vi "Pitstop.vi"(8 "Robot in":T1, 9 "robos":u32[](array[numeric]), 10 "IA State Input":T3={"our_robots"=[], "enemy_robots"=[], "balls"=[], "geometry"={"line_width"=0, "field_length"=0, "field_width"=0, "boundary_width"=0, "referee_width"=0, "goal_width"=0, "goal_depth"=0, "goal_wall_width"=0, "center_circle_radius"=0, "defense_radius"=0, "defense_stretch"=0, "free_kick_from_defense_dist"=0, "penalty_spot_from_field_line_dist"=0, "penalty_line_from_spot_dist"=0}, "IA Judge"={"stage"="", "command"="", "our_goalie_id"=0.0, "enemy_goalie_id"=0.0, "command\nenum"=enum."Halt", "Time"=enum."Azul"}, "Received Timestamp"=timestamp(0 s since 1904-01-01), "Events"={"Touch"=FALSE, "Ball out"=FALSE, "id touch"=0.0, "Ball out of \nVision"=FALSE, "Ball inside \nGoalie area"=FALSE, "Robot not responding"=FALSE, "Robots responding status"=[1.0, 1.0, 1.0, 1.0, 1.0, 1.0]}}) -> (1 "Robot out":T1)   [LabVIEW 2016]
uses:
  Core/AI Input.ctl
  Core/AI Robot.ctl
  Functions Enum.ctl
  Core/AI Ball.ctl
  Core/Field Size.ctl
  Core/AI Judge.ctl
  Command Enum.ctl
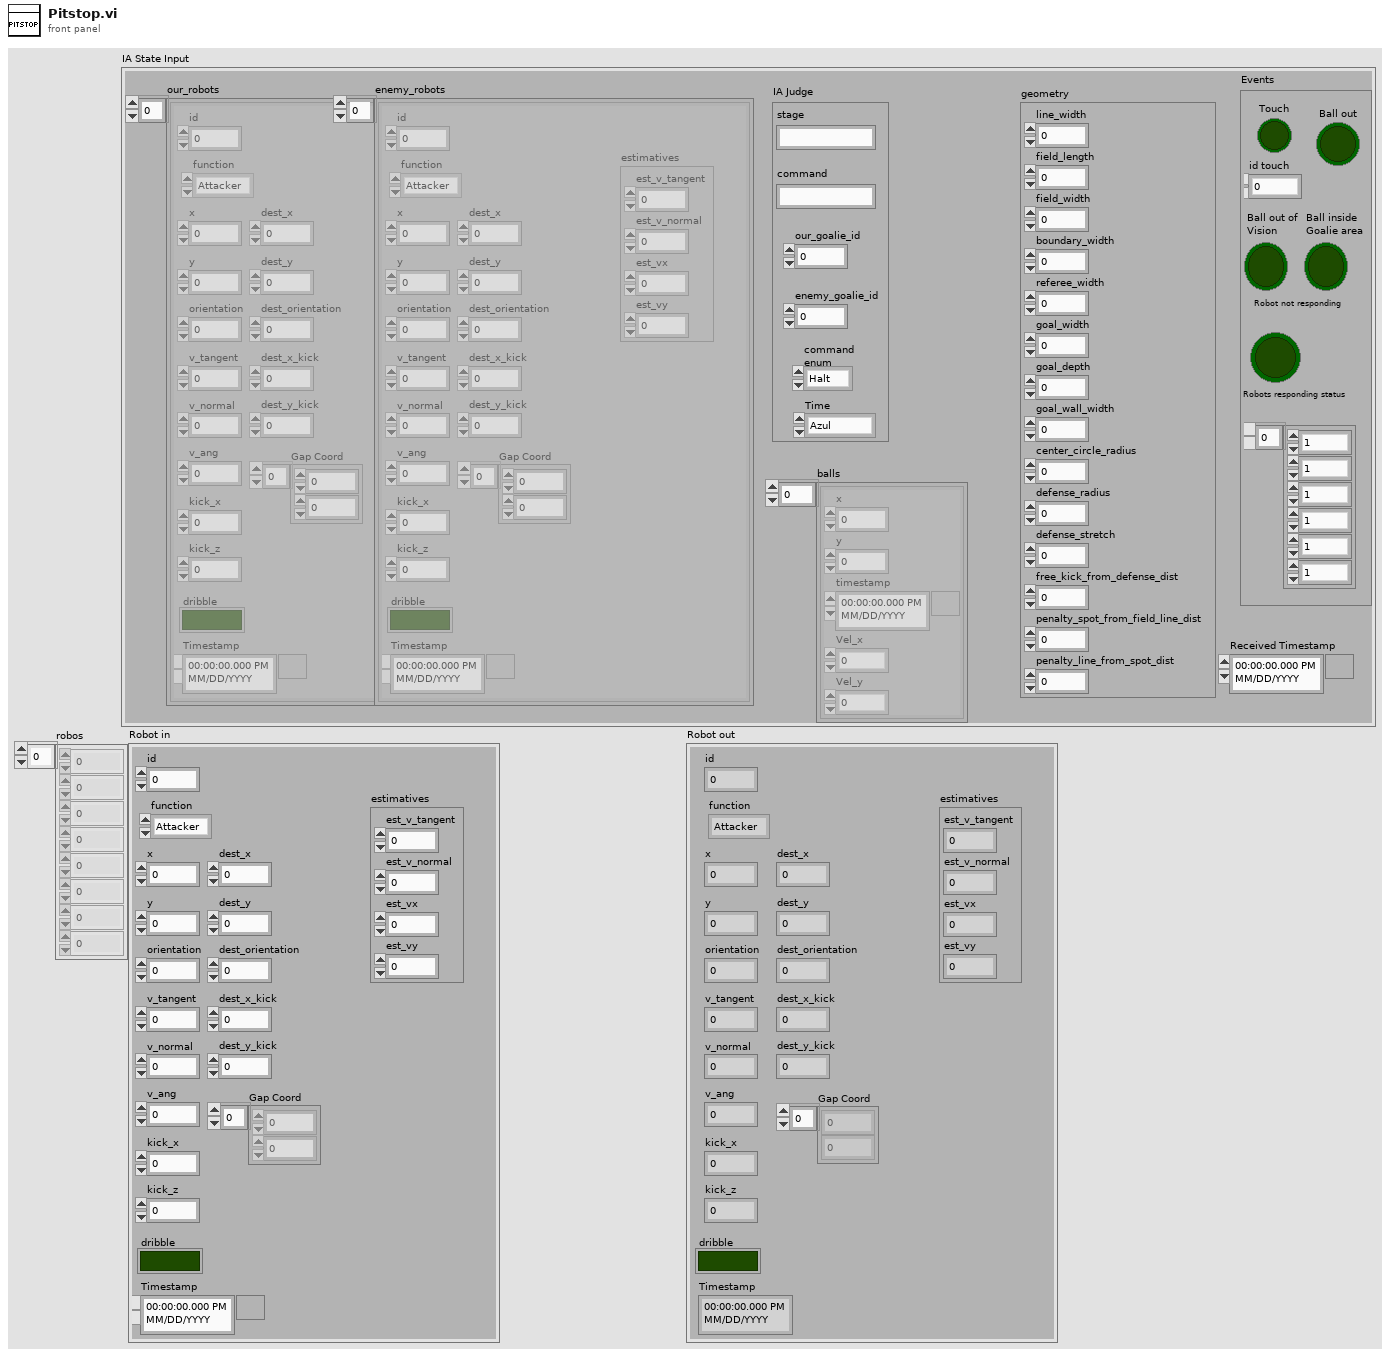
[diagram p1: front panel]
types:
  T1 = typedef "AI Robot.ctl" = cluster{"id":u32, "function":T2, "x":dbl, "y":dbl, "orientation":dbl, "v_tangent":dbl, "v_normal":dbl, "v_ang":dbl, "kick_x":dbl, "kick_z":dbl, "dribble":bool, "Timestamp":timestamp, "dest_x":dbl, "dest_y":dbl, "dest_orientation":dbl, "estimatives":cluster{"est_v_tangent":dbl, "est_v_normal":dbl, "est_vx":dbl, "est_vy":dbl}, "dest_x_kick":dbl, "dest_y_kick":dbl, "Gap Coord":dbl[]}
  T2 = typedef "Functions Enum.ctl" = enum16{"Attacker", "Goalie", "Defender", "Striker", "Goto 0", "Dummy", "Kicker", "ZigZag"}
  T3 = typedef "AI Input.ctl" = cluster{"our_robots":T1[], "enemy_robots":T1[], "balls":T4[], "geometry":T5, "IA Judge":T6, "Received Timestamp":timestamp, "Events":cluster{"Touch":bool, "Ball out":bool, "id touch":dbl, "Ball out of \nVision":bool, "Ball inside \nGoalie area":bool, "Robot not responding":bool, "Robots responding status":dbl[]}}
  T4 = typedef "AI Ball.ctl" = cluster{"x":dbl, "y":dbl, "timestamp":timestamp, "Vel_x":dbl, "Vel_y":dbl}
  T5 = typedef "Field Size.ctl" = cluster{"line_width":u32, "field_length":u32, "field_width":u32, "boundary_width":u32, "referee_width":u32, "goal_width":u32, "goal_depth":u32, "goal_wall_width":u32, "center_circle_radius":u32, "defense_radius":u32, "defense_stretch":u32, "free_kick_from_defense_dist":u32, "penalty_spot_from_field_line_dist":u32, "penalty_line_from_spot_dist":u32}
  T6 = typedef "AI Judge.ctl" = cluster{"stage":string, "command":string, "our_goalie_id":dbl, "enemy_goalie_id":dbl, "command\nenum":T7, "Time":enum16{"Azul", "Amarelo"}}
  T7 = typedef "Command Enum.ctl" = enum16{"Halt", "Stop", "Force Start", "PKA Normal Start", "Prepare Kickoff Ally", "PKE Normal Start", "Prepare Kickoff Enemy", "Prepare Penalty Ally", "PPA Normal Start", "Prepare Penalty Enemy", "PPE Normal Start", "Direct Free Enemy", "Direct Free Ally", "Indirect Free Enemy", "Indirect Free Ally", "Timeout Enemy", "Timeout Ally", "Goal Enemy", "Goal Ally", "Ball Placement Enemy", "Ball Placement Ally", "None"}
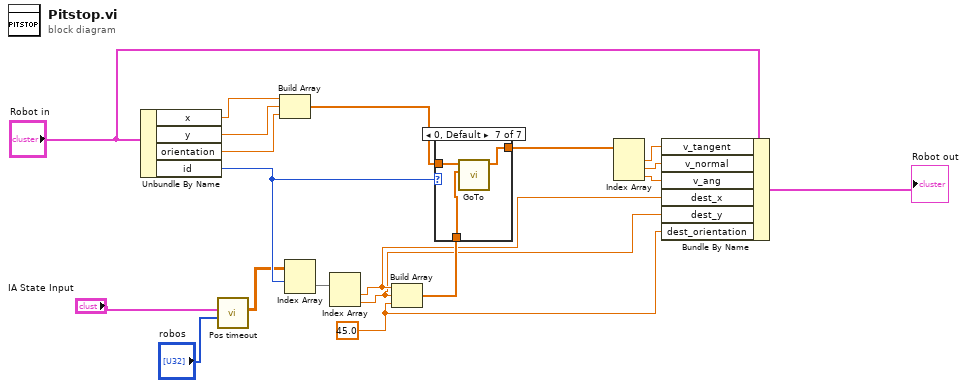
[diagram p0: block diagram]
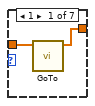
[diagram p2: hidden frame]
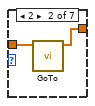
[diagram p3: hidden frame]
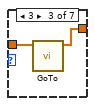
[diagram p4: hidden frame]
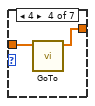
[diagram p5: hidden frame]
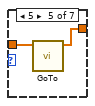
[diagram p6: hidden frame]
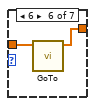
[diagram p7: hidden frame]
diagram:
  w4 = 45.0 ("element")
  n1 = Unbundle By Name("Robot in") -> ("x"=w17:dbl, "y"=w16:dbl, "orientation"=w15:dbl, "id"=w10:u32)
  n2 = call "Pos timeout.vi"("robos"="robos", "IA State Input"="IA State Input") -> ("Posição dos robos"=w9:dbl[][])  [unwired: 9 in]
  n3 = Build Array(w17, w16, w15) -> (w14:dbl[])
  n4 = Index Array(array=w9, index (row)=w10) -> (element=w8:dbl[])  [unwired: 1 in]
  n5 = Index Array(array=w8) -> (element #1=w6:dbl, element #2=w5:dbl)  [unwired: 2 in]
  n6 = Build Array(w6, w5, w4) -> (w7:dbl[])
  n7 = case shown="0, Default" w10 {
    tunnel: w14 -> [w21 w23 w25 w27 w29 w31 w34]
    tunnel: [w20 w22 w24 w26 w28 w30 w33] -> w18
    tunnel: w7 -> [_ _ _ _ _ _ w32]
    frame 1 {
      n8 = call "GoTo.vi"("Position"=w21) -> ("Output\nVelocity"=w20:dbl[])  [unwired: 9 in, 1 out]
    }
    frame 2 {
      n9 = call "GoTo.vi"("Position"=w23) -> ("Output\nVelocity"=w22:dbl[])  [unwired: 9 in, 1 out]
    }
    frame 3 {
      n10 = call "GoTo.vi"("Position"=w25) -> ("Output\nVelocity"=w24:dbl[])  [unwired: 9 in, 1 out]
    }
    frame 4 {
      n11 = call "GoTo.vi"("Position"=w27) -> ("Output\nVelocity"=w26:dbl[])  [unwired: 9 in, 1 out]
    }
    frame 5 {
      n12 = call "GoTo.vi"("Position"=w29) -> ("Output\nVelocity"=w28:dbl[])  [unwired: 9 in, 1 out]
    }
    frame 6 {
      n13 = call "GoTo.vi"("Position"=w31) -> ("Output\nVelocity"=w30:dbl[])  [unwired: 9 in, 1 out]
    }
    frame 0, Default {
      n14 = call "GoTo.vi"("Target"=w32, "Position"=w34) -> ("Output\nVelocity"=w33:dbl[])  [unwired: 8 in, 1 out]
    }
  }
  n15 = Index Array(array=w18) -> (element #1=w13:dbl, element #2=w12:dbl, element #3=w11:dbl)  [unwired: 3 in]
  n16 = Bundle By Name(cluster="Robot in", "v_tangent"=w13, "v_normal"=w12, "v_ang"=w11, "dest_x"=w6, "dest_y"=w5, "dest_orientation"=w4) -> (→"Robot out":T1)
